vi "TimingGenSGL_src.vi"(0 "Upercent":sgl caption="u voltage" format="%.21g", 1 "Period":u32, 5 "Vpercent":sgl caption="v voltage" format="%.21g", 7 "Wpercent":sgl caption="w voltage" format="%.21g") -> (4 "U_Timing":T1, 6 "V_Timing":T1, 8 "W_timing":T1)   [LabVIEW 2015]
uses:
  ON_OFF_timing.ctl
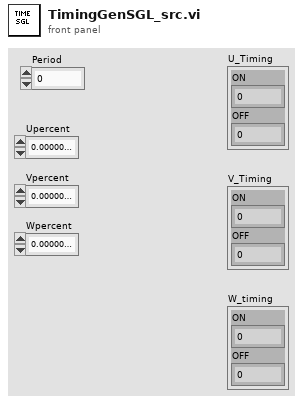
[diagram p1: front panel]
types:
  T1 = typedef "ON_OFF_timing.ctl" = cluster{"ON":u32, "OFF":u32}
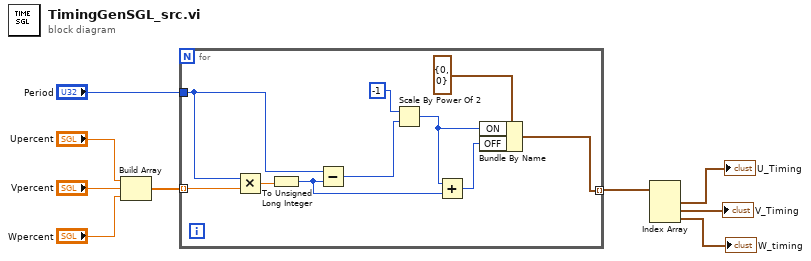
[diagram p0: block diagram]
diagram:
  n1 = Build Array("Upercent", "Vpercent", "Wpercent") -> (w6:sgl[])
  n2 = for {
    tunnel: w6 -> [w15] mode=indexing
    tunnel: "Period" -> [w14]
    tunnel: [w10] -> w4 mode=indexing
    n3 = Multiply(x=w14, y=w15) -> (x*y=w19:sgl)
    n4 = To Unsigned Long Integer(number=w19) -> (unsigned 32bit integer=w17:u32)
    n5 = Subtract(x=w14, y=w17) -> (x-y=w16:u32)
    n6 = Scale By Power Of 2(n=i16 -1, x=w16) -> (x*2^n=w12:u32)
    n7 = Add(x=w12, y=w17) -> (x+y=w11:u32)
    n8 = Bundle By Name(cluster=T1 {"ON"=0, "OFF"=0} ("ON_OFF"), "ON"=w12, "OFF"=w11) -> (w10:T1)
  }
  n9 = Index Array(array=w4) -> (element #1=→"U_Timing":T1, element #2=→"V_Timing":T1, element #3=→"W_timing":T1)  [unwired: 3 in]
